vi "Untitled 5.vi"   [LabVIEW 2013]
uses:
  <resource>/Framework/Providers/LVClassLibrary/NewAccessors/BaseAccessorScripter/BaseAccessorScripter.lvclass
  <resource>/Framework/Providers/LVClassLibrary/NewAccessors/CLSUIP_Access.ctl
  <resource>/Framework/Providers/LVClassLibrary/NewAccessors/MemberVICreation.lvlib
types:
  T1 = typedef "MemberVICreation.lvlib/CLSUIP_Access.ctl" = enum16{"Read", "Write", "R/W"}
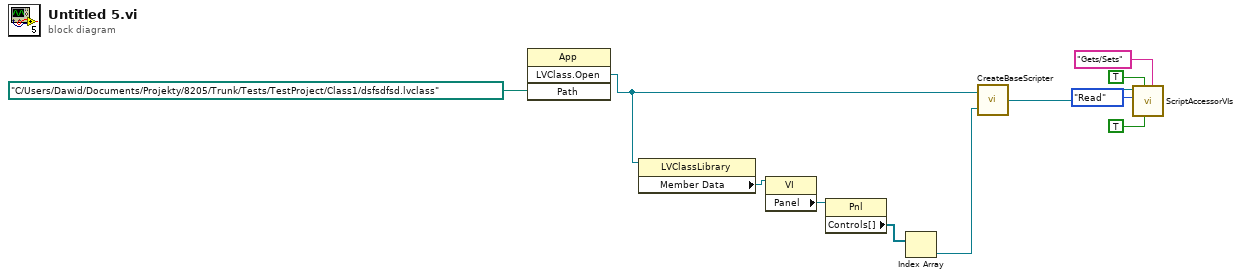
[diagram p0: block diagram]
diagram:
  n1 = invoke class="App" method="LVClass.Open"("Path"=path "C:/Users/Dawid/Documents/Projekty/8205/Trunk/Tests/TestProject/Class1/dsfsdfsd.lvclass" ("vi path")) -> ("LVClass.Open"=w6:refnum<vi>)  [unwired: 3 in, 3 out]
  n2 = property class="LVClassLibrary"(reference=w6) -> ("Member Data"=w9:refnum<vi>)  [unwired: 1 in, 2 out]
  n3 = property class="VI"(reference=w9) -> ("Panel"=w8:refnum<vi>)  [unwired: 1 in, 2 out]
  n4 = property class="Pnl"(reference=w8) -> ("Controls[]"=w7:refnum<vi>[])  [unwired: 1 in, 2 out]
  n5 = Index Array(array=w7) -> (element=w5:refnum<vi>)  [unwired: 1 in]
  n6 = call <resource>:"CreateBaseScripter.vi"("Ctl Refnum"=w5, "LVClassLibrary Ref"=w6) -> ("Scripter Out"=w11:refnum<class "BaseAccessorScripter.lvclass">)
  n7 = call-dynamic "ScriptAccessorVIs.vi"("Virtual Folder Name"="Gets/Sets", "Create as Properties"=TRUE, "Include error terminals"=TRUE, "Access"=CLSUIP_Access."Read", "BaseAccessorScripter in"=w11) -> ()  [unwired: 5 in, 2 out]
